vi "Handle Message.vi"(6 "Acknowledge Data":T1, 8 "error in (no error)":errorcluster, 9 "Module Action":string, 10 "Message Data Out":variant, 11 "Module Data In":refnum<class "Rename.lvclass">) -> (0 "error out":errorcluster, 1 "Module Action":string, 2 "Stop Module":bool, 3 "Module Data Out":refnum<class "Rename.lvclass">, 4 "Acknowledge Data":T1)   [LabVIEW 2015, in "Generic Module Library.lvlib" / "Template G_Module.lvlib"]
uses:
  Template G_Module.lvlib
  Module Class/Rename.lvclass
  Private Controls/Module Message Cluster Components/Acknowledge Data Cluster.ctl
  Private Controls/Module Message Cluster Components/Ack Payload.ctl
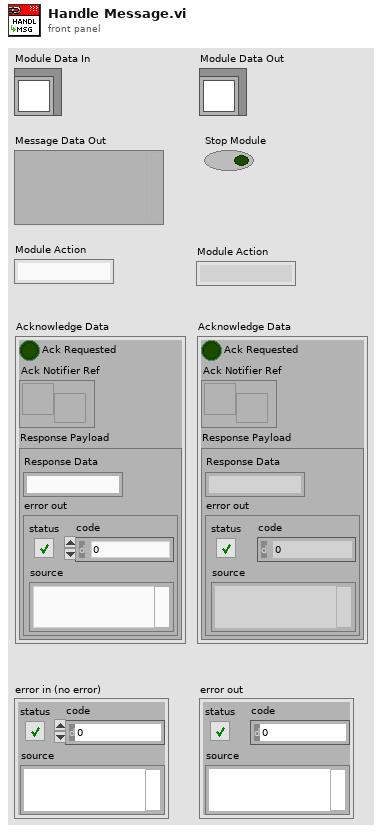
[diagram p1: front panel]
types:
  T1 = typedef "Generic Module Library.lvlib/Template G_Module.lvlib/Acknowledge Data Cluster.ctl" = cluster{"Ack Requested":bool, "Ack Notifier Ref":refnum<notifier>, "Response Payload":T2}
  T2 = typedef "Generic Module Library.lvlib/Template G_Module.lvlib/Ack Payload.ctl" = cluster{"Response Data":string, "error out":errorcluster}
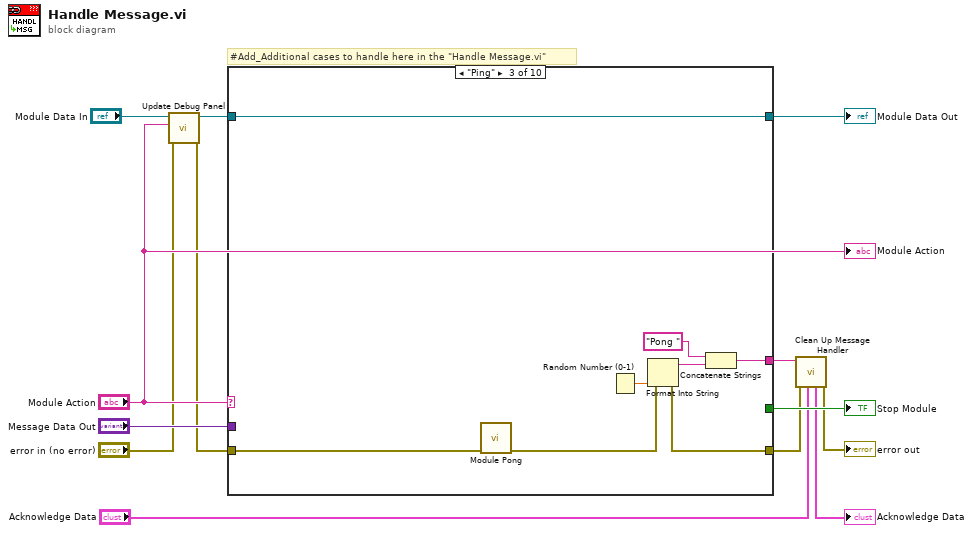
[diagram p0: block diagram]
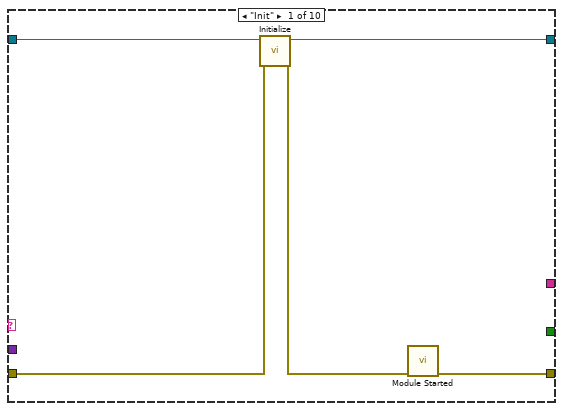
[diagram p2: hidden frame]
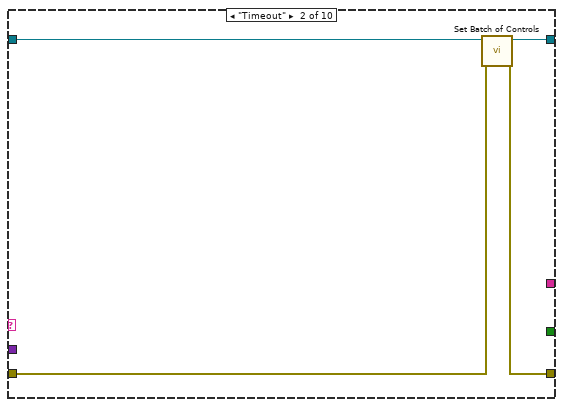
[diagram p3: hidden frame]
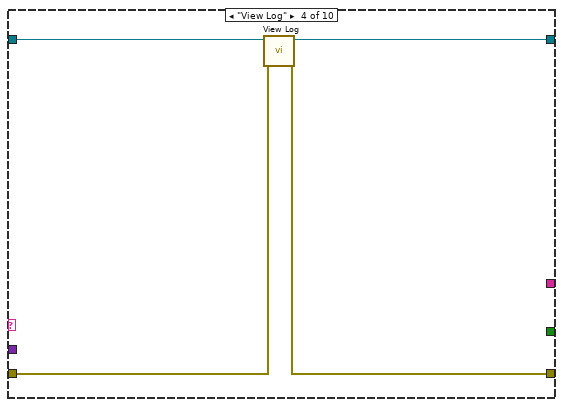
[diagram p4: hidden frame]
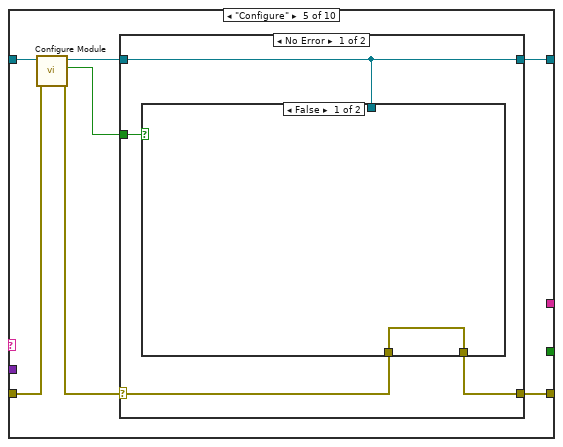
[diagram p5: hidden frame]
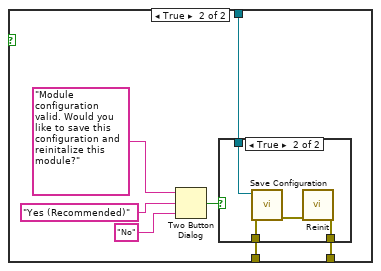
[diagram p6: hidden frame]
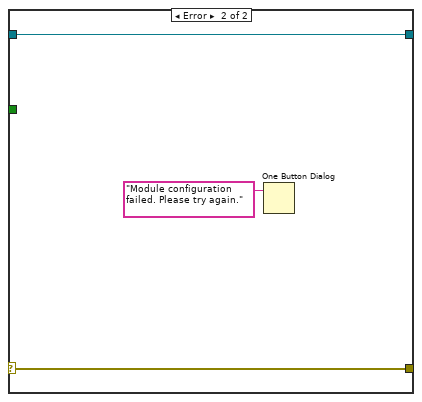
[diagram p8: hidden frame]
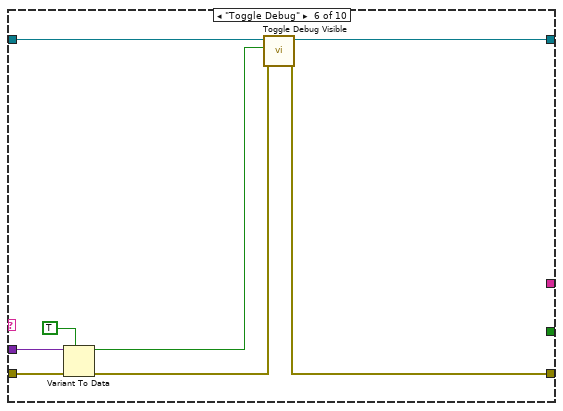
[diagram p9: hidden frame]
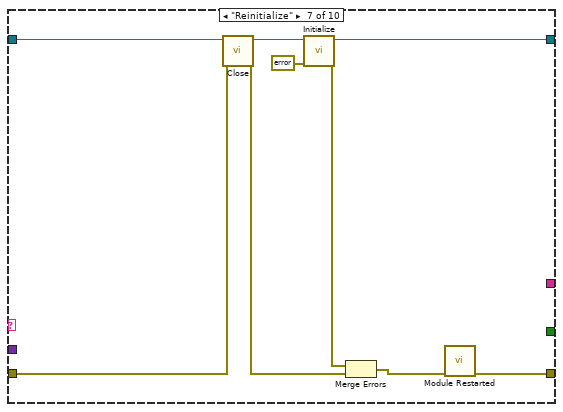
[diagram p10: hidden frame]
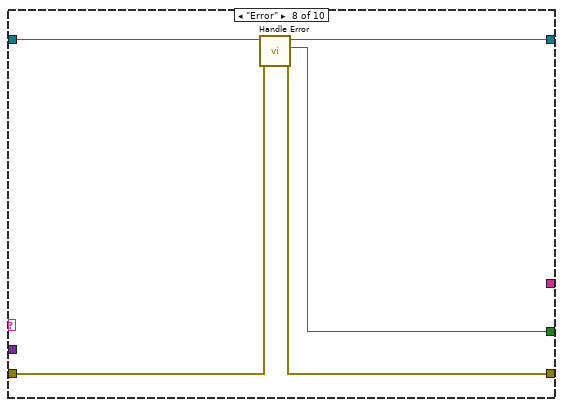
[diagram p11: hidden frame]
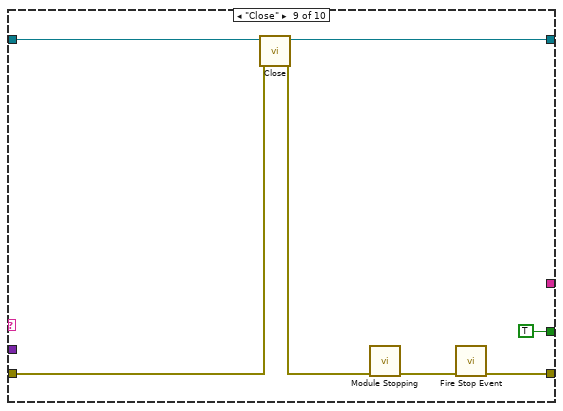
[diagram p12: hidden frame]
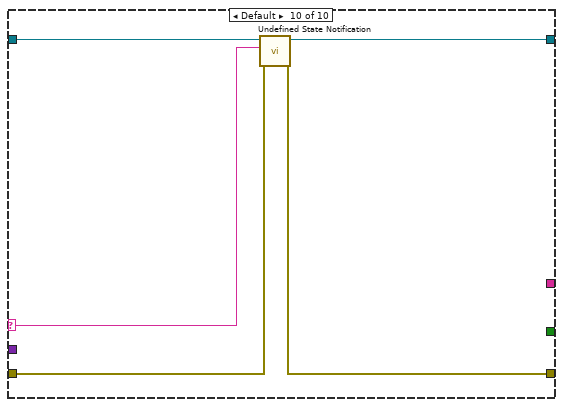
[diagram p13: hidden frame]
diagram:
  # "#Add_Additional cases to handle here in the \"Handle Message.vi\""
  n1 = call "Update Debug Panel.vi"("error in (no error)"="error in (no error)", "Module Action"="Module Action", "Rename in"="Module Data In") -> ("error out"=w1:errorcluster, "Rename out"=w5:refnum<class "Rename.lvclass">)  [unwired: 7 in]
  n2 = case shown="\"Ping\"" "Module Action" {
    selector: "Module Action" -> [_ _ _ _ _ _ _ _ _ w91]
    tunnel: w5 -> [w18 w21 w30 w34 w36 w68 w73 w82 w88 w95]
    tunnel: [w17 w22 w30 w33 w38 w69 w74 w83 w87 w94] -> w13
    tunnel: w1 -> [w16 w19 w29 w32 w41 w67 w72 w81 w86 w93]
    tunnel: [w14 w20 w25 w31 w40 w66 w70 w80 w89 w92] -> w9
    tunnel: [_ _ _ _ _ _ _ w79 TRUE _] -> w11
    tunnel: "Message Data Out" -> [_ _ _ _ _ w64 _ _ _ _]
    tunnel: [_ _ w24 _ _ _ _ _ _ _] -> w10
    frame "Init" {
      n3 = call-dynamic "Initialize.vi"("error in (no error)"=w16, "Module Data In"=w18) -> ("error out"=w15:errorcluster, "Module Data Out"=w17:refnum<class "Rename.lvclass">)  [unwired: 8 in]
      n4 = call "Module Started.vi"("error in"=w15) -> ("error out"=w14:errorcluster)  [unwired: 10 in]
    }
    frame "Timeout" {
      n5 = call "Set Batch of Controls.vi"("error in (no error)"=w19, "Rename in"=w21) -> ("error out"=w20:errorcluster, "Rename out"=w22:refnum<class "Rename.lvclass">)  [unwired: 8 in]
    }
    frame "Ping" {
      n6 = call "Module Pong.vi"("error in"=w29) -> ("error out"=w26:errorcluster)  [unwired: 10 in]
      n7 = Random Number (0-1)() -> (number: 0 to 1=w27:dbl)
      n8 = Format Into String(error in=w26, w27) -> (resulting string=w28:string, error out=w25:errorcluster)  [unwired: 2 in]
      n9 = Concatenate Strings("Pong " ("string"), w28) -> (w24:string)
    }
    frame "View Log" {
      n10 = call "View Log.vi"("error in (no error)"=w32, "Rename in"=w34) -> ("error out"=w31:errorcluster, "Rename out"=w33:refnum<class "Rename.lvclass">)  [unwired: 8 in]
    }
    frame "Configure" {
      n11 = call "Configure Module.vi"("error in (no error)"=w41, "Rename in"=w36) -> ("error out"=w39:errorcluster, "Changed"=w35:bool, "Rename out"=w37:refnum<class "Rename.lvclass">)  [unwired: 7 in]
      n12 = case shown="No Error" w39 {
        selector: w39 -> [w44 w61]
        tunnel: [w45 w61] -> w40
        tunnel: w37 -> [w43 w59]
        tunnel: [w43 w59] -> w38
        tunnel: w35 -> [w42 _]
        frame No Error {
          n13 = case shown="False" w42 {
            tunnel: [w46 w53] -> w45
            tunnel: w44 -> [w46 w48]
            tunnel: w43 -> [_ w47]
            frame False {
            }
            frame True {
              n14 = Two Button Dialog(message="Module configuration valid. Would you like to save this configuration and reinitalize this module?", 1:"No" ("F button name (\"Cancel\")"), 2:"Yes (Recommended)" ("T button name (\"OK\")")) -> (T button?=w49:bool)
              n15 = case shown="True" w49 {
                tunnel: [w54 w58] -> w53
                tunnel: w47 -> [_ w57]
                tunnel: w48 -> [w54 w56]
                frame False {
                }
                frame True {
                  n16 = call "Save Configuration.vi"("error in"=w56, "Module Data"=w57) -> ("error out"=w55:errorcluster)  [unwired: 9 in]
                  n17 = call "Reinit.vi"("error in"=w55) -> ("error out"=w58:errorcluster)  [unwired: 10 in]
                }
              }
            }
          }
        }
        frame Error {
          n18 = One Button Dialog(message="Module configuration failed. Please try again.") -> ()  [unwired: 1 in, 1 out]
        }
      }
    }
    frame "Toggle Debug" {
      n19 = Variant To Data(error in=w67, type=TRUE, Variant=w64) -> (data=w62:bool, error out=w65:errorcluster)
      n20 = call "Toggle Debug Visible.vi"("error in (no error)"=w65, "Visible"=w62, "Rename in"=w68) -> ("error out"=w66:errorcluster, "Rename out"=w69:refnum<class "Rename.lvclass">)  [unwired: 7 in]
    }
    frame "Reinitialize" {
      n21 = call-dynamic "Close.vi"("error in (no error)"=w72, "Module Data In"=w73) -> ("error out"=w78:errorcluster, "Module Data Out"=w77:refnum<class "Rename.lvclass">)  [unwired: 8 in]
      n22 = call-dynamic "Initialize.vi"("error in (no error)"=errorcluster {"status"=FALSE, "code"=0, "source"=""}, "Module Data In"=w77) -> ("error out"=w76:errorcluster, "Module Data Out"=w74:refnum<class "Rename.lvclass">)  [unwired: 8 in]
      n23 = Merge Errors(w76, w78) -> (w71:errorcluster)
      n24 = call "Module Restarted.vi"("error in"=w71) -> ("error out"=w70:errorcluster)  [unwired: 10 in]
    }
    frame "Error" {
      n25 = call-dynamic "Handle Error.vi"("error in (no error)"=w81, "Module Data In"=w82) -> ("error out"=w80:errorcluster, "Stop Module"=w79:bool, "Module Data Out"=w83:refnum<class "Rename.lvclass">)  [unwired: 7 in]
    }
    frame "Close" {
      n26 = call-dynamic "Close.vi"("error in (no error)"=w86, "Module Data In"=w88) -> ("error out"=w85:errorcluster, "Module Data Out"=w87:refnum<class "Rename.lvclass">)  [unwired: 8 in]
      n27 = call "Module Stopping.vi"("error in"=w85) -> ("error out"=w84:errorcluster)  [unwired: 10 in]
      n28 = call "Fire Stop Event.vi"("error in"=w84) -> ("error out"=w89:errorcluster)  [unwired: 10 in]
    }
    frame Default {
      n29 = call-dynamic "Undefined State Notification.vi"("error in"=w93, "Undefined state"=w91, "Rename in"=w95) -> ("error out"=w92:errorcluster, "Rename out"=w94:refnum<class "Rename.lvclass">)  [unwired: 7 in]
    }
  }
  "Module Data Out" <- w13
  "Stop Module" <- w11
  n30 = call "Clean Up Message Handler.vi"("Acknowledge Data in"="Acknowledge Data", "error in"=w9, "Response String"=w10) -> ("error out"=→"error out":errorcluster, "Acknowledge Data out"=→"Acknowledge Data":T1)  [unwired: 7 in]
  "Module Action" <- "Module Action"
